vi "times2Delays.vi"(8 "error in (no error)":errorcluster, 10 "data":dbl[][][](array[numeric]), 11 "K2602 in":refnum<class "K2602.lvclass">) -> (0 "error out":errorcluster, 2 "data out":dbl[][][](array[numeric]), 3 "K2602 out":refnum<class "K2602.lvclass">)   [LabVIEW 2011, in "Hardware.lvlib" / "Channels.lvlib" / "K2602.lvclass"]
uses:
  K2602.lvclass
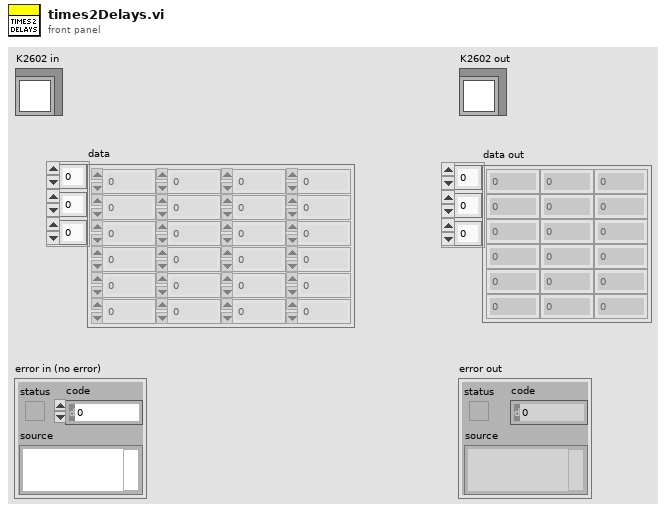
[diagram p1: front panel]
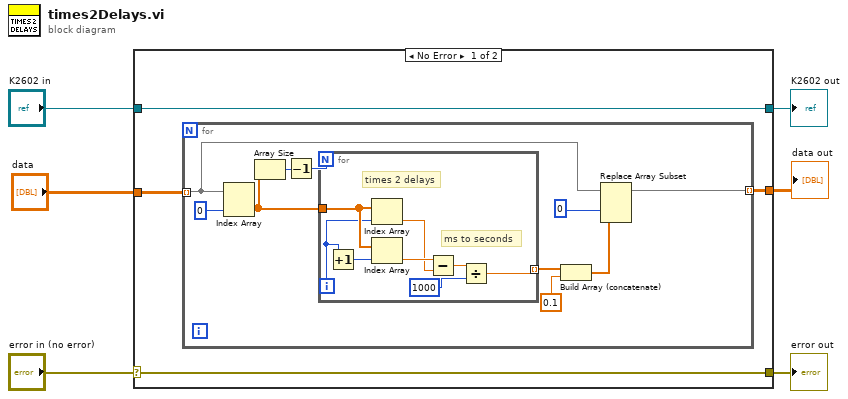
[diagram p0: block diagram]
diagram:
  n1 = case shown="No Error" "error in (no error)" {
    selector: "error in (no error)" -> [w9 w30]
    tunnel: [w9 w30] -> w5
    tunnel: [w10 w29] -> w3
    tunnel: "K2602 in" -> [w10 w29]
    tunnel: "data" -> [w8 _]
    tunnel: [w7 _] -> w1
    frame No Error {
      n2 = for {
        tunnel: w8 -> [w16] mode=indexing
        tunnel: [w14] -> w7 mode=indexing
        n3 = Index Array(array=w16, index (col)=0) -> (element=w17:dbl[])  [unwired: 1 in]
        n4 = Array Size(array=w17) -> (size(s)=w18:i32)
        n5 = Decrement(x=w18) -> (x-1=w19:i32)
        n6 = for {
          N: w19 -> [_]
          tunnel: w17 -> [w28]
          tunnel: [w22] -> w13 mode=indexing
          i -> [w27]
          # "times 2 delays"
          # "ms to seconds"
          n7 = Increment(x=w27) -> (x+1=w26:i32)
          n8 = Index Array(array=w28, index=w27) -> (element=w24:dbl)
          n9 = Index Array(array=w28, index=w26) -> (element=w25:dbl)
          n10 = Subtract(x=w25, y=w24) -> (x-y=w23:dbl)
          n11 = Divide(x=w23, y=1000) -> (x/y=w22:dbl)
        }
        n12 = Build Array (concatenate)(w13, 0.1) -> (w11:dbl[])
        n13 = Replace Array Subset(array=w16, new element=w11, index (col)=0) -> (w14:dbl[][])  [unwired: 1 in]
      }
    }
    frame Error {
    }
  }
  "error out" <- w5
  "K2602 out" <- w3
  "data out" <- w1
